vi "Points_Generator.vi"(6 "Частота (1000 Hz)":dbl, 7 "Время между импульсами, с in":dbl, 8 "Коэффициент амплитуды":dbl, 9 "Ширина отрицательного импульса, с in":dbl, 10 "Количество точек in":dbl, 11 "Ширина импульса, с in":dbl=1000.0) -> (0 "Общее количество точек":dbl, 1 "Количество точек, до начала второго импульса, тчк":dbl, 2 "Ширина двух импульсов, тчк":dbl, 3 "Ширина одног импульса, тчк":dbl, 4 "Два импульса (детектер)":i32[](array[numeric]), 5 "Один импульс (диод)":dbl[](array[numeric]))   [LabVIEW 2012]
panel:
  out "Оставшиеся точки":string
  out "Начало второго импульса":string
  out "Начало интервала":string
  out "Количество точек":string caption="String"
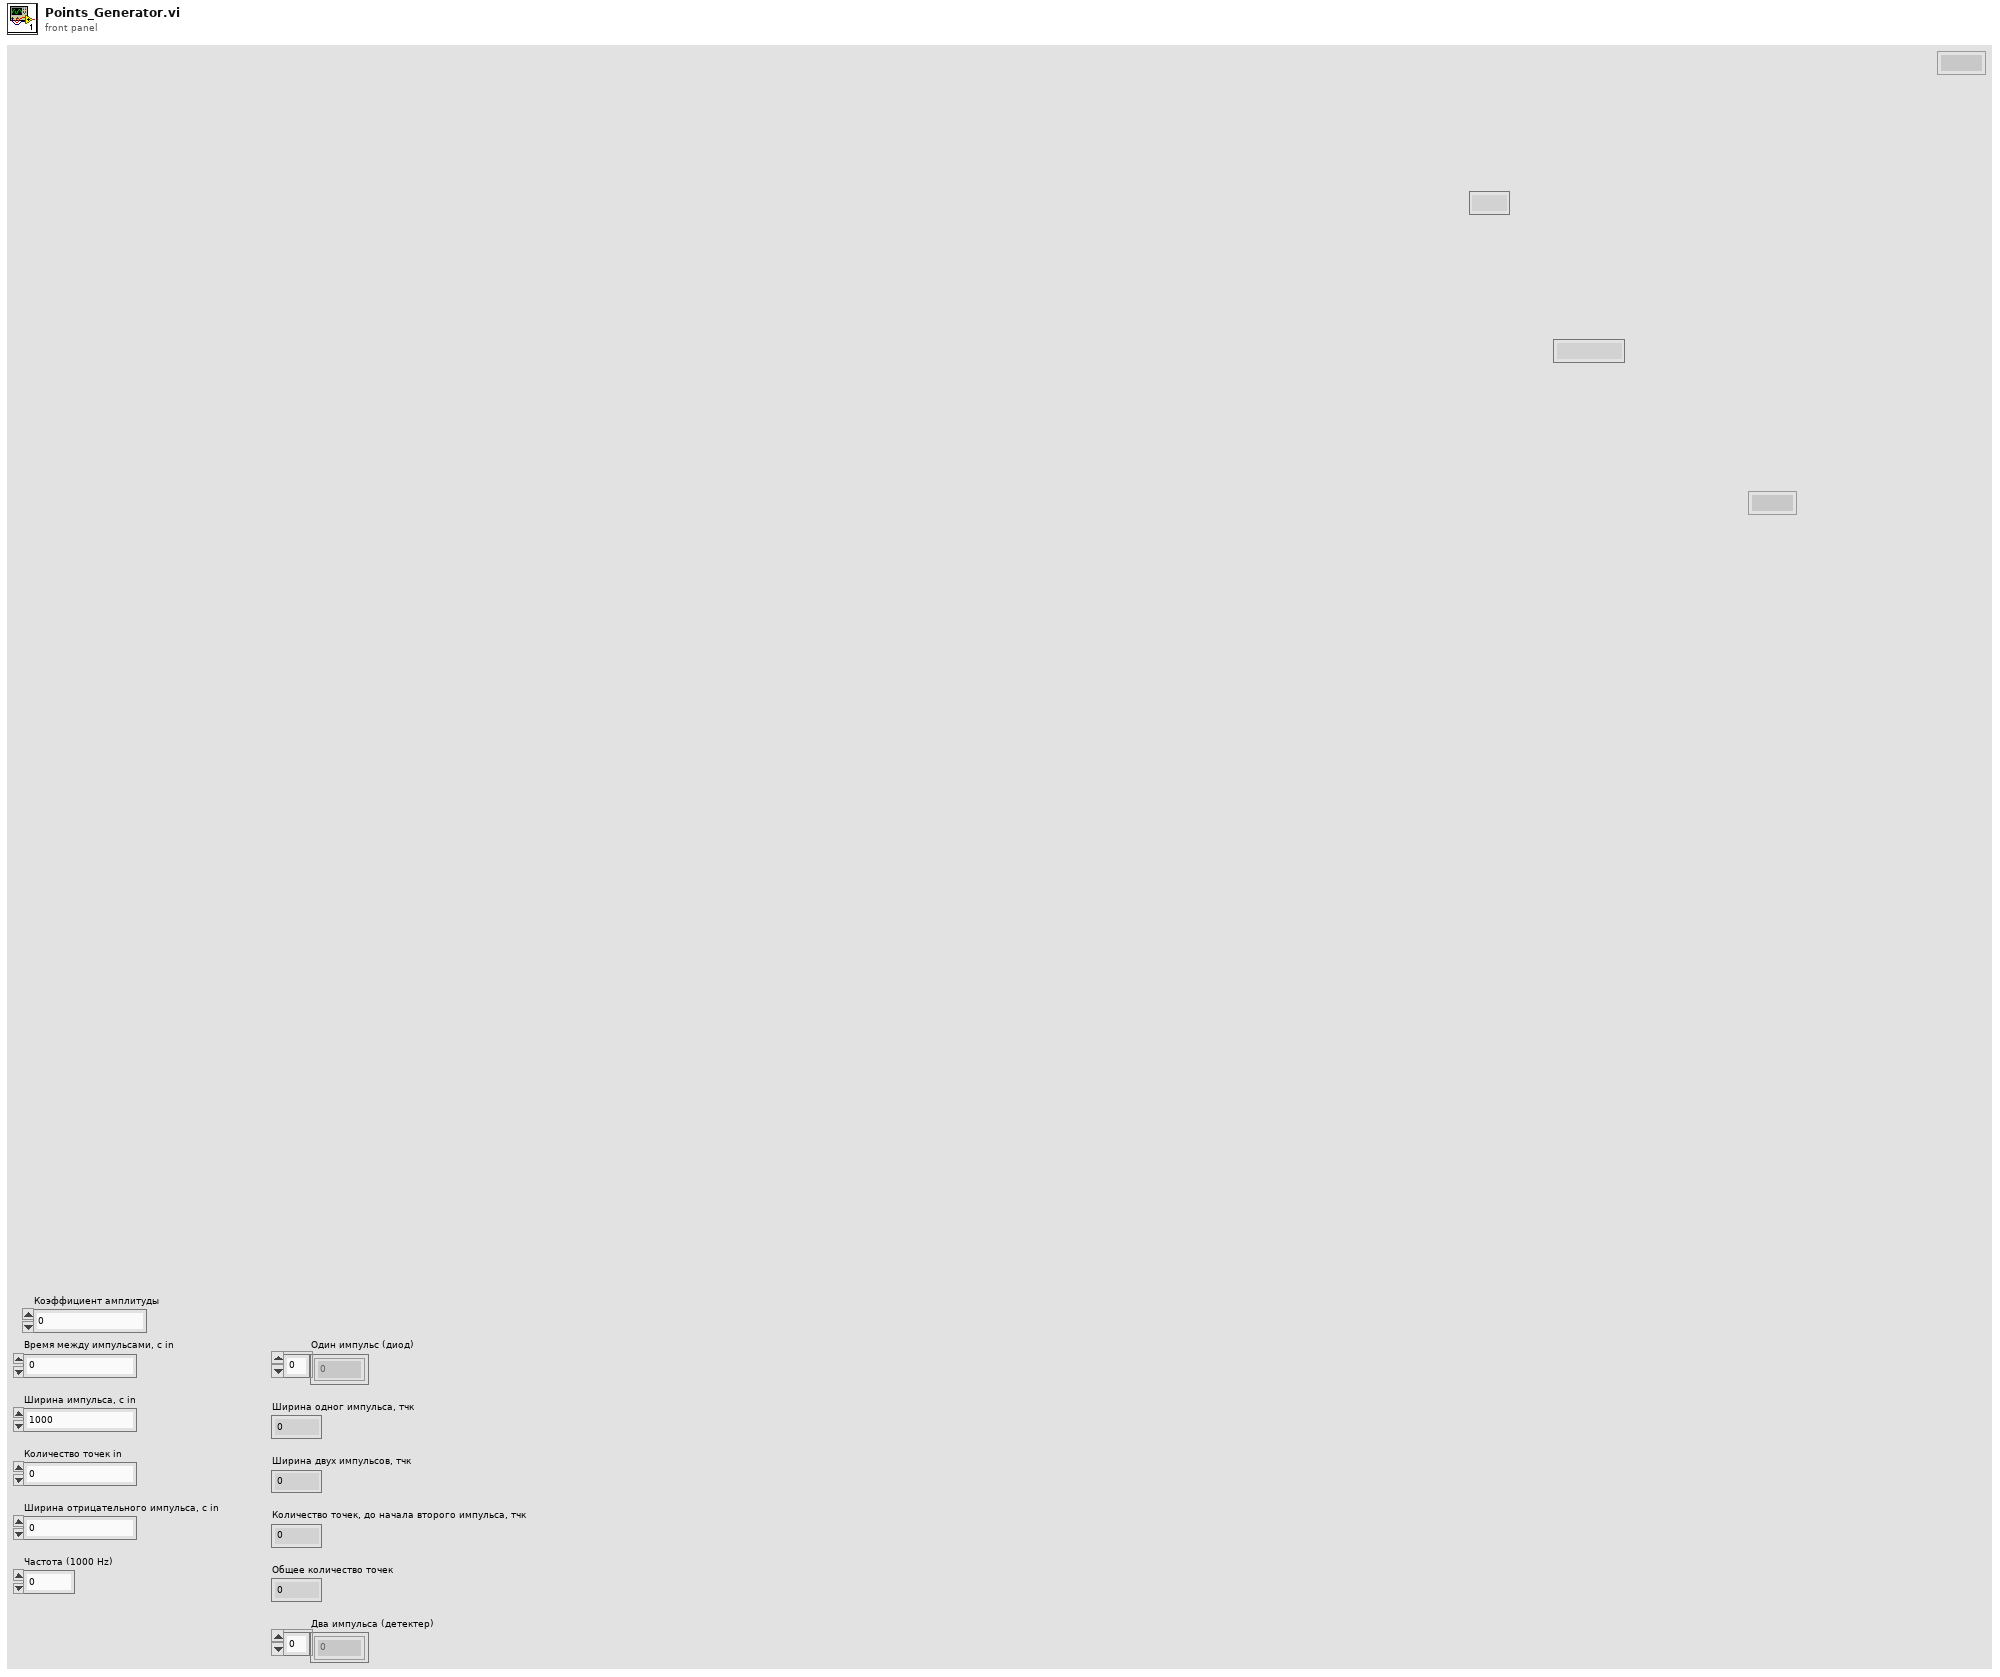
[diagram p1: front panel]
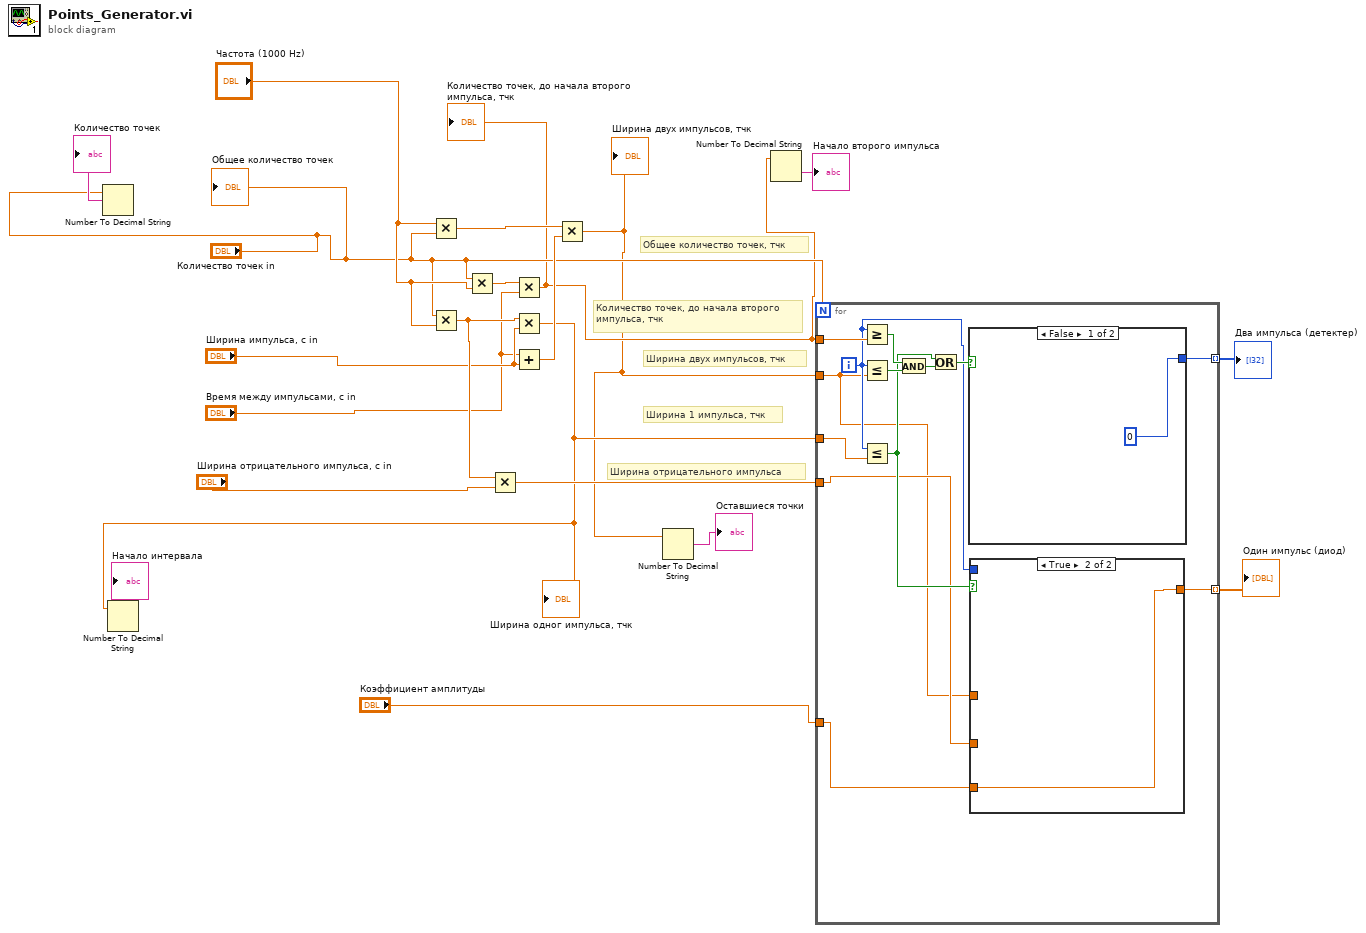
[diagram p0: block diagram]
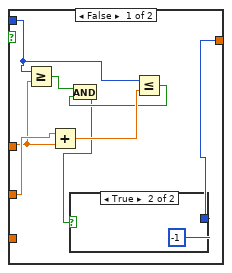
[diagram p2: hidden frame]
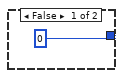
[diagram p3: hidden frame]
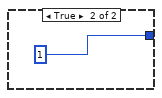
[diagram p4: hidden frame]
diagram:
  # "Ширина отрицательного импульса"
  # "Общее количество точек, тчк"
  # "Количество точек, до начала второго импульса, тчк"
  # "Ширина двух импульсов, тчк"
  # "Ширина 1 импульса, тчк"
  n1 = Number To Decimal String(number="Количество точек in") -> (decimal integer string=→"Количество точек":string)  [unwired: 1 in]
  n2 = Multiply(x="Частота (1000 Hz)", y="Количество точек in") -> (x*y=w15:dbl)
  n3 = Multiply(x="Количество точек in", y="Частота (1000 Hz)") -> (x*y=w18:dbl)
  n4 = Multiply(x="Количество точек in", y="Частота (1000 Hz)") -> (x*y=w14:dbl)
  n5 = Multiply(x=w18, y="Ширина отрицательного импульса, с in") -> (x*y=w20:dbl)
  n6 = Multiply(x=w14, y="Время между импульсами, с in") -> (x*y=w5:dbl)
  "Количество точек, до начала второго импульса, тчк" <- w5
  n7 = Multiply(x=w18, y="Ширина импульса, с in") -> (x*y=w7:dbl)
  "Ширина одног импульса, тчк" <- w7
  n8 = Number To Decimal String(number=w7) -> (decimal integer string=→"Начало интервала":string)  [unwired: 1 in]
  n9 = Add(x="Время между импульсами, с in", y="Ширина импульса, с in") -> (x+y=w16:dbl)
  n10 = Multiply(x=w15, y=w16) -> (x*y=w3:dbl)
  "Ширина двух импульсов, тчк" <- w3
  n11 = Number To Decimal String(number=w3) -> (decimal integer string=→"Оставшиеся точки":string)  [unwired: 1 in]
  n12 = Number To Decimal String(number=w5) -> (decimal integer string=→"Начало второго импульса":string)  [unwired: 1 in]
  n13 = for {
    N: "Количество точек in" -> [_]
    tunnel: [w33] -> w12 mode=indexing
    tunnel: w7 -> [w32]
    tunnel: w5 -> [w27]
    tunnel: w3 -> [w22]
    tunnel: [w25] -> w13 mode=indexing
    tunnel: w20 -> [w24]
    tunnel: "Коэффициент амплитуды" -> [w21]
    i -> [w23]
    n14 = Greater Or Equal?(x=w23, y=w27) -> (x >= y?=w29:bool)
    n15 = Less Or Equal?(x=w23, y=w22) -> (x <= y?=w28:bool)
    n16 = Less Or Equal?(x=w23, y=w32) -> (x <= y?=w26:bool)
    n17 = And(x=w29, y=w28) -> (x .and. y?=w31:bool)
    n18 = Or(x=w26, y=w31) -> (x .or. y?=w30:bool)
    n19 = case shown="False" w30 {
      tunnel: [0 1] -> w33
      frame False {
      }
      frame True {
      }
    }
    n20 = case shown="True" w26 {
      tunnel: [w37 w44] -> w25
      tunnel: w24 -> [w36 _]
      tunnel: w23 -> [w35 _]
      tunnel: w22 -> [w34 _]
      tunnel: w21 -> [_ w44]
      frame False {
        n21 = Greater Or Equal?(x=w35, y=w34) -> (x >= y?=w40:bool)
        n22 = Add(x=w36, y=w34) -> (x+y=w41:dbl)
        n23 = Less Or Equal?(x=w35, y=w41) -> (x <= y?=w39:bool)
        n24 = And(x=w40, y=w39) -> (x .and. y?=w38:bool)
        n25 = case shown="True" w38 {
          tunnel: [0 -1] -> w37
          frame False {
          }
          frame True {
          }
        }
      }
      frame True {
      }
    }
  }
  "Один импульс (диод)" <- w13
  "Два импульса (детектер)" <- w12
  "Общее количество точек" <- "Количество точек in"
